vi "z motion pattern_v2.vi"(9 "traj array size":i32, 10 "no of lobes":i8, 11 "Window Array":dbl[](array[numeric])) -> (2 "-sin(n_flr*s).*w":dbl[](array[numeric]), 3 "-sin(n_flr*s)":dbl[](array[numeric]))   [LabVIEW 2010]
uses:
  <vilib>/Analysis/NI_AALBase.lvlib
  <vilib>/Analysis/1siggen.llb/Ramp Pattern by Samples.vi
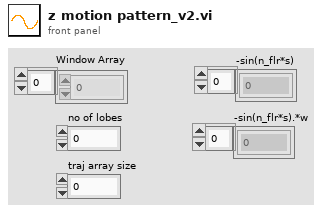
[diagram p1: front panel]
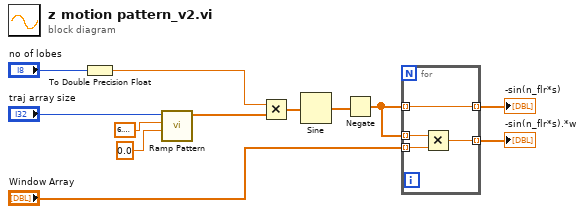
[diagram p0: block diagram]
diagram:
  n1 = To Double Precision Float(number="no of lobes") -> (double precision float=w5:dbl)
  n2 = call-poly <vilib>:"Ramp Pattern.vi"("start"=0.0, "end"=6.283185307179586, "samples"="traj array size") -> ("Ramp Pattern"=w8:dbl[])  [unwired: 7 in, 1 out]
  n3 = Multiply(x=w5, y=w8) -> (x*y=w2:dbl[])
  n4 = Sine(x=w2) -> (sin(x)=w1:dbl[])
  n5 = Negate(x=w1) -> (-x=w3:dbl[])
  n6 = for {
    tunnel: "Window Array" -> [w15] mode=indexing
    tunnel: [w16] -> w6 mode=indexing
    tunnel: w3 -> [w14] mode=indexing
    tunnel: [w13] -> w4 mode=indexing
    tunnel: w3 -> [w13] mode=indexing
    n7 = Multiply(x=w14, y=w15) -> (x*y=w16:dbl)
  }
  "-sin(n_flr*s).*w" <- w6
  "-sin(n_flr*s)" <- w4
